vi "QueryTimingAndSyncHardware.vi"(8 "error in (no error)":errorcluster, 11 "Chassis Reference in":refnum<k24>) -> (0 "error out":errorcluster, 2 "Devices out":string[](array[string]), 3 "Chassis Reference out":refnum<k24>)   [LabVIEW 2015, in "VeriStandTestUtilities.lvlib"]
uses:
  VeriStandTestUtilities.lvlib
  NationalInstruments.VeriStand.SystemDefinitionAPI
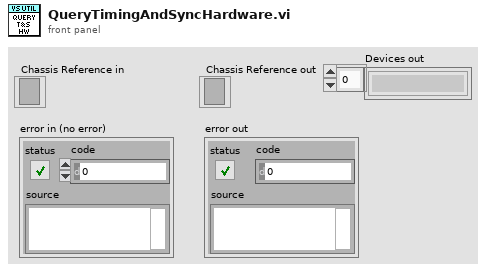
[diagram p1: front panel]
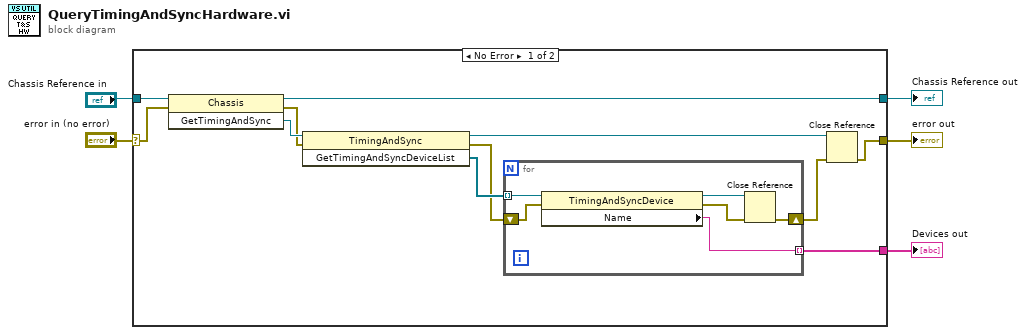
[diagram p0: block diagram]
diagram:
  n1 = case shown="No Error" "error in (no error)" {
    selector: "error in (no error)" -> [w14 w23]
    tunnel: [w10 w23] -> w5
    tunnel: [w16 w24] -> w4
    tunnel: "Chassis Reference in" -> [w15 w24]
    tunnel: [w6 _] -> w1
    frame No Error {
      n2 = invoke class="Chassis" method="GetTimingAndSync"(reference=w15, error in=w14) -> (reference out=w16:refnum<k24>, error out=w12:errorcluster, "GetTimingAndSync"=w13:refnum<k24>)  [unwired: 1 in]
      n3 = invoke class="TimingAndSync" method="GetTimingAndSyncDeviceList"(reference=w13, error in=w12) -> (reference out=w11:refnum<k24>, error out=w7:errorcluster, "GetTimingAndSyncDeviceList"=w9:refnum<k24>[])  [unwired: 1 in]
      n4 = for {
        tunnel: w9 -> [w22] mode=indexing
        shift-right: [w21] -> w8
        shift-left: w7 -> [w19]
        tunnel: [w17] -> w6 mode=indexing
        n5 = property class="TimingAndSyncDevice"(reference=w22, error in=w19) -> (reference out=w20:refnum<k24>, error out=w18:errorcluster, "Name"=w17:string)
        n6 = Close Reference(reference=w20, error in (no error)=w18) -> (error out=w21:errorcluster)
      }
      n7 = Close Reference(reference=w11, error in (no error)=w8) -> (error out=w10:errorcluster)
    }
    frame Error {
    }
  }
  "error out" <- w5
  "Chassis Reference out" <- w4
  "Devices out" <- w1
